vi "Settings Dialog.vi"(8 "error in (no error)":errorcluster, 11 "Settings in":T2={"Hardware Configuration"={"VISA Refnum in"="", "Serial Configuration"={"Baud Rate"=460800, "Flow Control"=0}, "Voltage Level (0V)"=0.0, "Output Phase(s) (1-Phase)"=0, "Active Phase (1:Phase 1)"=1}, "Logging Configuration"={"Log File Base Path"=path "", "TDMS File Reference"=refnum}} {"Hardware Configuration"."Output Phase(s) (1-Phase)" items=["3 phase", "1 phase"]; "Hardware Configuration"."Active Phase (1:Phase 1)" items=["Phase 1"=1, "Phase 2"=2, "Phase 3"=3]; "Hardware Configuration"."Serial Configuration"."Flow Control" items=["None", "XON/XOFF", "RTS/CTS", "XON/XOFF & RTS/CTS", "DTR/DSR", "XON/XOFF & DTR/DSR"]; "Hardware Configuration"."Serial Configuration"."Baud Rate" items=["9600"=9600, "19200"=19200, "38400"=38400, "57600"=57600, "115200"=115200, "230400"=230400, "460800"=460800]}) -> (0 "error out":errorcluster, 1 "Cancelled?":bool, 2 "UI Refresh Needed?":bool, 3 "Settings out":T2={"Hardware Configuration"={"VISA Refnum in"="", "Serial Configuration"={"Baud Rate"=460800, "Flow Control"=0}, "Voltage Level (0V)"=0.0, "Output Phase(s) (1-Phase)"=0, "Active Phase (1:Phase 1)"=1}, "Logging Configuration"={"Log File Base Path"=path "", "TDMS File Reference"=refnum}} {"Hardware Configuration"."Output Phase(s) (1-Phase)" items=["3 phase", "1 phase"]; "Hardware Configuration"."Active Phase (1:Phase 1)" items=["Phase 1"=1, "Phase 2"=2, "Phase 3"=3]; "Hardware Configuration"."Serial Configuration"."Flow Control" items=["None", "XON/XOFF", "RTS/CTS", "XON/XOFF & RTS/CTS", "DTR/DSR", "XON/XOFF & DTR/DSR"]; "Hardware Configuration"."Serial Configuration"."Baud Rate" items=["9600"=9600, "19200"=19200, "38400"=38400, "57600"=57600, "115200"=115200, "230400"=230400, "460800"=460800]})   [LabVIEW 2013, in "Cal Inst Settings.lvlib"]
doc: "Dialog for selecting user specified settings."
uses:
  Cal Inst Settings.lvlib
  Settings.ctl
  Acquisition/Hardware Configuration.ctl
  Logging/Logging Configuration.ctl
  <vilib>/Utility/xml.llb/Write to XML File(string).vi
  Acquisition/Cal Inst Acquisition.lvlib
  Logging/Cal Inst Logging.lvlib
panel:
  in  "Hardware Configuration":T1={"VISA Refnum in"="", "Serial Configuration"={"Baud Rate"=460800, "Flow Control"=0}, "Voltage Level (0V)"=0.0, "Output Phase(s) (1-Phase)"=0, "Active Phase (1:Phase 1)"=1} {"Output Phase(s) (1-Phase)" items=["3 phase", "1 phase"]; "Active Phase (1:Phase 1)" items=["Phase 1"=1, "Phase 2"=2, "Phase 3"=3]; "Serial Configuration"."Flow Control" items=["None", "XON/XOFF", "RTS/CTS", "XON/XOFF & RTS/CTS", "DTR/DSR", "XON/XOFF & DTR/DSR"]; "Serial Configuration"."Baud Rate" items=["9600"=9600, "19200"=19200, "38400"=38400, "57600"=57600, "115200"=115200, "230400"=230400, "460800"=460800]}
  in  "Log File Path":path=path "C:/Users/dhstuart/Dropbox/CLTC/CaliforniaInstrumentsIxSeries/Output"
  in  "Cancel Button":bool
  in  "OK Button":bool
  # "Non visible portion of dialog (needed for connector pane)."
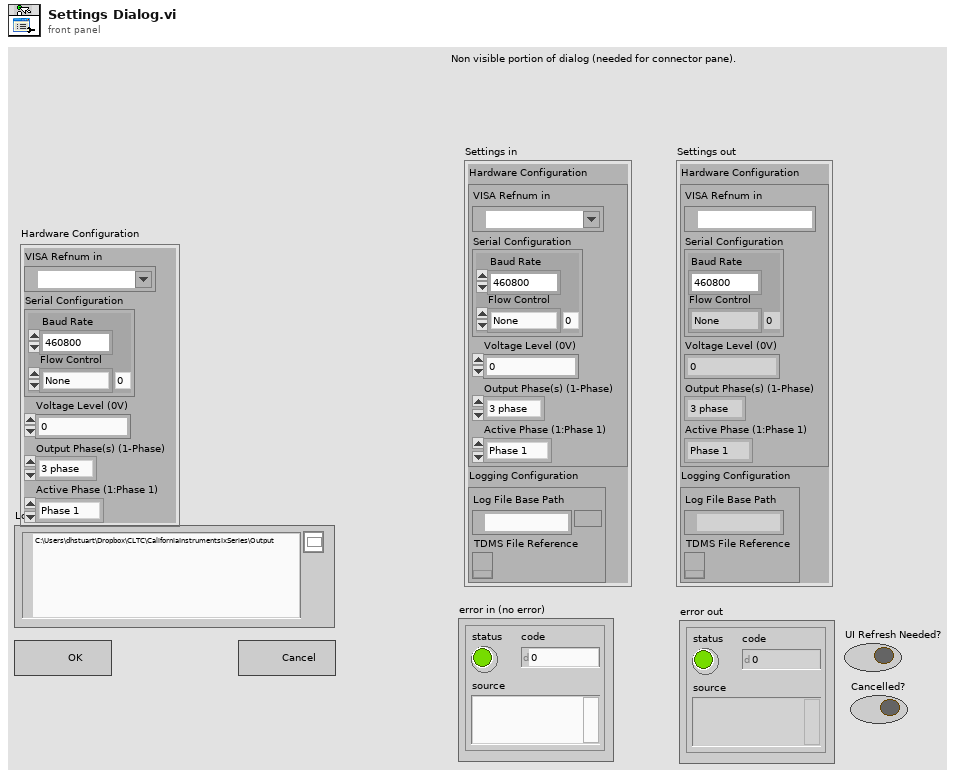
[diagram p1: front panel]
types:
  T1 = typedef "Cal Inst Acquisition.lvlib/Hardware Configuration.ctl" = cluster{"VISA Refnum in":refnum<visa-resource-name>, "Serial Configuration":cluster{"Baud Rate":u32, "Flow Control":u16}, "Voltage Level (0V)":dbl, "Output Phase(s) (1-Phase)":u16, "Active Phase (1:Phase 1)":i32}
  T2 = typedef "Cal Inst Settings.lvlib/Settings.ctl" = cluster{"Hardware Configuration":T1, "Logging Configuration":T3}
  T3 = typedef "Cal Inst Logging.lvlib/Logging Configuration.ctl" = cluster{"Log File Base Path":path, "TDMS File Reference":refnum<k34>}
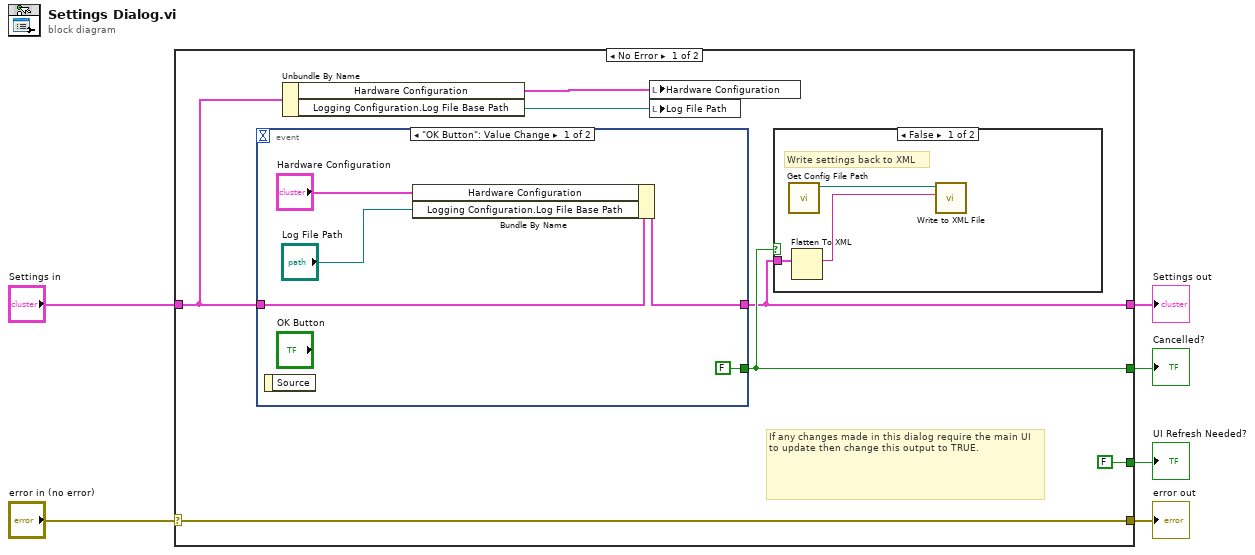
[diagram p0: block diagram]
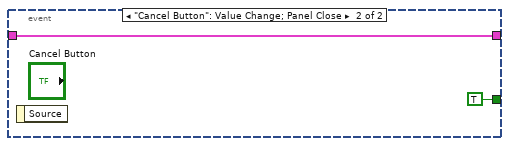
[diagram p3: hidden frame]
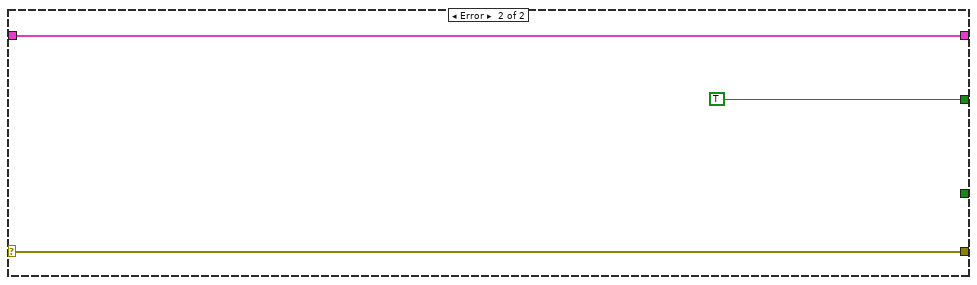
[diagram p4: hidden frame]
diagram:
  n1 = case shown="No Error" "error in (no error)" {
    selector: "error in (no error)" -> [w13 w26]
    tunnel: [w13 w26] -> w5
    tunnel: "Settings in" -> [w9 w25]
    tunnel: [w10 w25] -> w3
    tunnel: [FALSE ("UI Refresh Needed?") _] -> w2
    tunnel: [w11 TRUE ("UI Refresh Needed?")] -> w1
    frame No Error {
      # "If any changes made in this dialog require the main UI to update then change this output to TRUE."
      n2 = event shown="[0] \"OK Button\": Value Change" {
        selector: _ -> [_ _]
        dyn-events: _ -> [_ _]
        timeout: _ -> [_ _]
        tunnel: [w19 w23] -> w10
        tunnel: w9 -> [w20 w23]
        tunnel: [FALSE ("UI Refresh Needed?") TRUE ("UI Refresh Needed?")] -> w11
        event "OK Button": Value Change {
          n3 = event-data() -> ()  [unwired: 1 in, 1 out]
          n4 = Bundle By Name(cluster=w20, "Hardware Configuration"="Hardware Configuration", "Logging Configuration.Log File Base Path"="Log File Path") -> (w19:T2)
        }
        event "Cancel Button": Value Change; Panel Close {
          n5 = event-data() -> ()  [unwired: 1 in, 1 out]
        }
      }
      n6 = Unbundle By Name(w9) -> ("Hardware Configuration"=w7:T1, "Logging Configuration.Log File Base Path"=w8:path)
      n7 = local write "Hardware Configuration"(w7) -> ()
      n8 = local write "Log File Path"(w8) -> ()
      n9 = case shown="False" w11 {
        tunnel: w10 -> [w15 _]
        frame False {
          # "Write settings back to XML"
          n10 = call "Get Config File Path.vi"() -> ("XML File Path"=w16:path)  [unwired: 10 in, 1 out]
          n11 = Flatten To XML(anything=w15) -> (xml string=w14:string)
          n12 = call-poly <vilib>:"Write to XML File.vi"("XML Input"=w14, "XML File Path"=w16) -> ()  [unwired: 7 in, 3 out]
        }
        frame True {
        }
      }
    }
    frame Error {
    }
  }
  "UI Refresh Needed?" <- w2
  "error out" <- w5
  "Settings out" <- w3
  "Cancelled?" <- w1
